vi "168xBReadVoltage_Current.vi"() -> ()   [LabVIEW 2015]
uses:
  <vilib>/Instr/_visa.llb/VISA Configure Serial Port (Instr).vi
panel:
  out "Current":dbl
  out "Voltage":dbl
  in  "VISA resource name":refnum<visa-resource-name>="COM5"
  out "read buffer":string
  out "error out":errorcluster
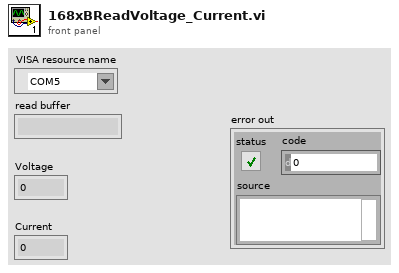
[diagram p1: front panel]
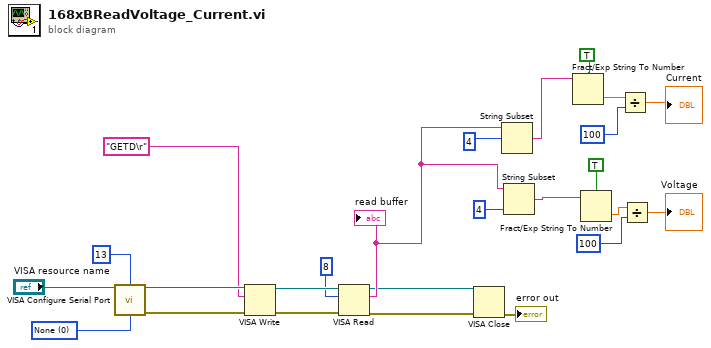
[diagram p0: block diagram]
diagram:
  w23 = u16 0 items=["None", "XON/XOFF", "RTS/CTS", "XON/XOFF & RTS/CTS", "DTR/DSR", "XON/XOFF & DTR/DSR"] ("flow control (0:none)")
  n1 = call-poly "VISA Configure Serial Port"("VISA resource name"="VISA resource name", "termination char\n(0xA = '\\n' = LF)"=u8 13 ("termination char\n(0xA = '\\n' = LF)"), "flow control (0:none)"=w23) -> ("VISA resource name out"=w18:refnum<visa-resource-name>, "error out"=w17:errorcluster)  [unwired: 11 in]
  n2 = VISA Write(VISA resource name=w18, write buffer="GETD\r", error in (no error)=w17) -> (VISA resource name out=w21:refnum<visa-resource-name>, error out=w22:errorcluster)  [unwired: 1 out]
  n3 = VISA Read(VISA resource name=w21, byte count=u32 8, error in (no error)=w22) -> (VISA resource name out=w2:refnum<visa-resource-name>, read buffer=w14:string, error out=w1:errorcluster)  [unwired: 1 out]
  "read buffer" <- w14
  n4 = VISA Close(VISA resource name=w2, error in (no error)=w1) -> (error out=→"error out":errorcluster)
  n5 = String Subset(string=w14, offset (0)=4) -> (substring=w10:string)  [unwired: 1 in]
  n6 = String Subset(string=w14, length (rest)=4) -> (substring=w9:string)  [unwired: 1 in]
  n7 = Fract/Exp String To Number(use system decimal point (T)=TRUE, string=w10) -> (number=w6:dbl)  [unwired: 2 in, 1 out]
  n8 = Fract/Exp String To Number(use system decimal point (T)=TRUE, string=w9) -> (number=w5:dbl)  [unwired: 2 in, 1 out]
  n9 = Divide(x=w6, y=100) -> (x/y=→"Current":dbl)
  n10 = Divide(x=w5, y=100) -> (x/y=→"Voltage":dbl)
